vi "FindCoordSys-2Rects.vi"() -> ()   [LabVIEW 2016]
uses:
  <vilib>/vision/Measure.llb/Edge Options.ctl
  <vilib>/vision/Measure.llb/Edge Polarity.ctl
  <vilib>/vision/NI_Vision_Development_Module.lvlib
panel:
  in  "Options":T3={"Direction"=0, "Primary Edge Options"={"Edge Polarity"=0, "Kernel Size"=3, "Width"=3, "Minimum Edge Strength"=10.0, "Interpolation Type"=enum."Bilinear Fixed", "Data Processing Method"=enum."Average"}, "Secondary Edge Options"={"Edge Polarity"=0, "Kernel Size"=3, "Width"=3, "Minimum Edge Strength"=10.0, "Interpolation Type"=enum."Bilinear Fixed", "Data Processing Method"=enum."Average"}, "Show Search Area"=TRUE, "Show Search Lines"=TRUE, "Show Edges Found"=TRUE, "Show Result"=TRUE, "Search Area Color"=65280, "Search Lines Color"=255, "Edge Locations Color"=16776960, "Result Color"=16711680, "Overlay Group Name"=""} {"Primary Edge Options"."Edge Polarity" items=["All Edges", "Rising Edges", "Falling Edges"]; "Primary Edge Options"."Minimum Edge Strength" format="%.2f"; "Primary Edge Options"."Width" step=2; "Primary Edge Options"."Kernel Size" step=2; "Secondary Edge Options"."Edge Polarity" items=["All Edges", "Rising Edges", "Falling Edges"]; "Secondary Edge Options"."Minimum Edge Strength" format="%.2f"; "Secondary Edge Options"."Width" step=2; "Secondary Edge Options"."Kernel Size" step=2}
  in  "Rectangle2":T4={"Left"=167, "Top"=134, "Right"=240, "Bottom"=218, "Rotation"=0.0} {"Rotation" min=-90.0 max=90.0 step=1.0 format="%.2f"; "Left" scale=0.0..1024.0; "Right" scale=0.0..1024.0}
  in  "Rectangle":T4={"Left"=50, "Top"=106, "Right"=150, "Bottom"=140, "Rotation"=0.0} {"Rotation" min=-90.0 max=90.0 step=1.0 format="%.2f"; "Left" scale=0.0..1024.0; "Right" scale=0.0..1024.0}
  out "Image":T5(plugin-control)
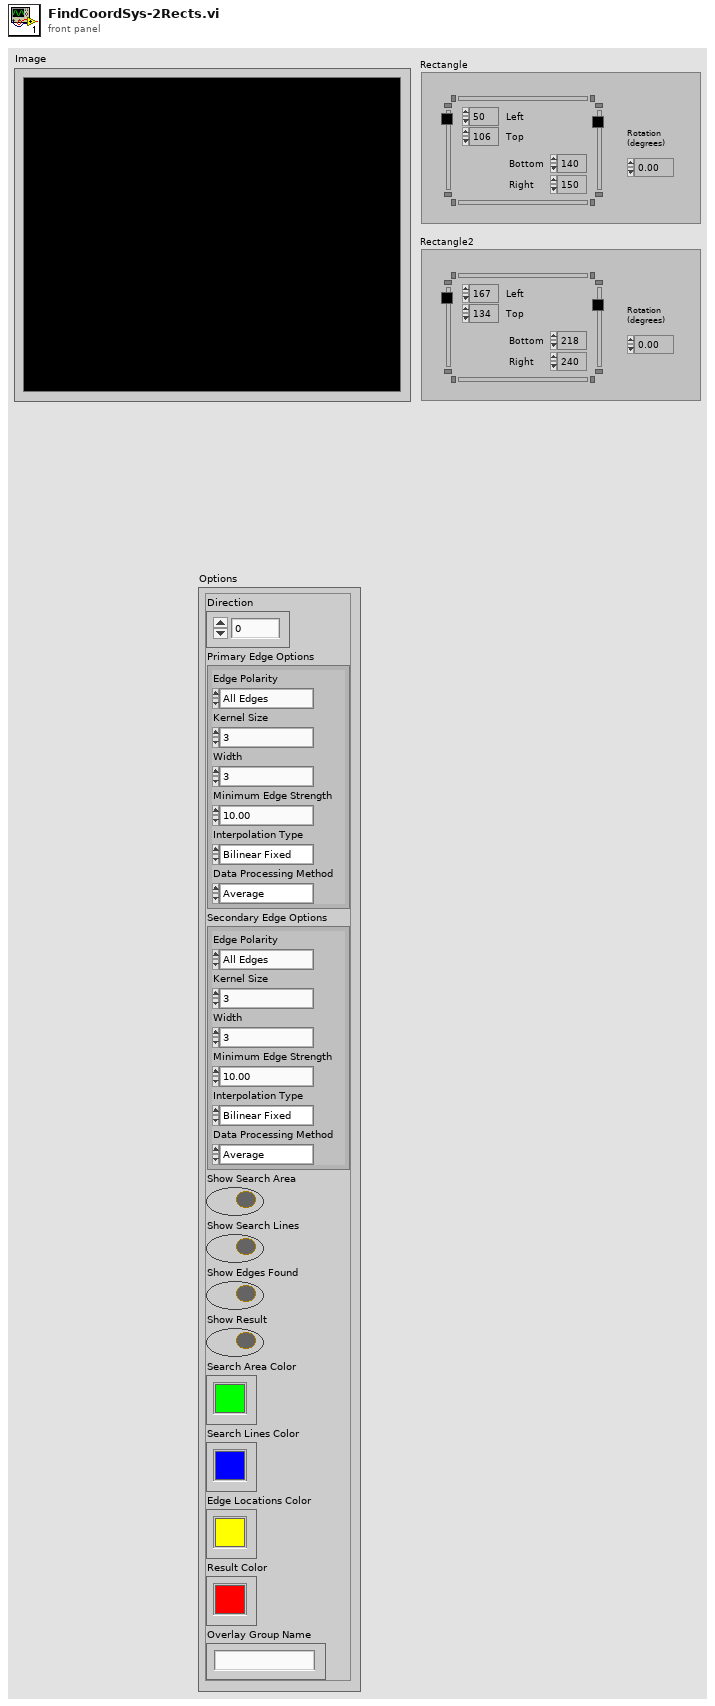
[diagram p1: front panel]
types:
  T1 = typedef "Edge Options.ctl" = cluster{"Edge Polarity":T2, "Kernel Size":u32, "Width":u32, "Minimum Edge Strength":sgl, "Interpolation Type":enum32{"Zero Order", "Bilinear", "Quadratic", "Cubic", "Bilinear Fixed"}, "Data Processing Method":enum32{"Average", "Median"}}
  T2 = typedef "Edge Polarity.ctl" = u32
  T3 = cluster{"Direction":u16, "Primary Edge Options":T1, "Secondary Edge Options":T1, "Show Search Area":bool, "Show Search Lines":bool, "Show Edges Found":bool, "Show Result":bool, "Search Area Color":u32, "Search Lines Color":u32, "Edge Locations Color":u32, "Result Color":u32, "Overlay Group Name":string}
  T4 = typedef "IMAQ Rectangle" = cluster{"Left":i32, "Top":i32, "Right":i32, "Bottom":i32, "Rotation":dbl}
  T5 = typedef "IMAQ Image.ctl" = refnum<image>
  T6 = typedef "ROI Descriptor" = cluster{"Global Rectangle":i32[], "Contours":cluster{"ID":enum32{"External", "Internal"}, "Type":u32, "Coordinates":i32[]}[]}
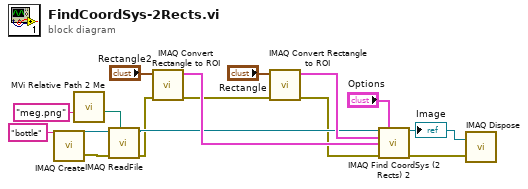
[diagram p0: block diagram]
diagram:
  n1 = call "IMAQ Create"("Image Name"="bottle") -> ("Src"=w7:T5, "error out"=w8:errorcluster)  [unwired: 4 in]
  n2 = call "MVi Relative Path 2 Me.vi"("Relative Path"="meg.png" ("Image Name")) -> ("Appended Dir"=w6:path)  [unwired: 5 in, 1 out]
  n3 = call "IMAQ ReadFile"("File Path"=w6, "error in (no error)"=w8, "Image"=w7) -> ("error out"=w3:errorcluster, "Image Out"=w5:T5)  [unwired: 4 in, 3 out]
  n4 = call "IMAQ Convert Rectangle to ROI"("error in (no error)"=w3, "Rectangle"="Rectangle2") -> ("error out"=w4:errorcluster, "ROI Descriptor"=w10:T6)  [unwired: 7 in]
  n5 = call "IMAQ Convert Rectangle to ROI"("error in (no error)"=w4, "Rectangle"="Rectangle") -> ("error out"=w2:errorcluster, "ROI Descriptor"=w13:T6)  [unwired: 7 in]
  n6 = call "IMAQ Find CoordSys (2 Rects) 2"("Image"=w5, "Options"="Options", "Primary ROI Descriptor"=w13, "Secondary ROI Descriptor"=w10, "error in (no error)"=w2) -> ("Image Out"=w15:T5, "error out"=w16:errorcluster)  [unwired: 6 in, 3 out]
  "Image" <- w15
  n7 = call "IMAQ Dispose"("Image"=w15, "error in (no error)"=w16) -> ()  [unwired: 4 in, 1 out]
